vi "Is Air Pocket Part of Exterior Air Way.vi"(4 "Lava Droplets":set{cluster{"X":i32, "Y":i32, "Z":i32}}(c389), 5 "Extreme Planes":cluster{"X":i32[], "Y":i32[], "Z":i32[]}, 6 "Possible Directions":cluster{"X":i32, "Y":i32, "Z":i32}[](array[cluster]), 7 "Air Pockets Connected to Exterior Surface in":set{cluster{"X":i32, "Y":i32, "Z":i32}}(c389), 9 "Locations in Search in":set{cluster{"X":i32, "Y":i32, "Z":i32}}(c389), 10 "Location":cluster{"X":i32, "Y":i32, "Z":i32}) -> (0 "Air Pockets Connected to Exterior Surface out":set{cluster{"X":i32, "Y":i32, "Z":i32}}(c389), 2 "Locations in Search out":set{cluster{"X":i32, "Y":i32, "Z":i32}}(c389), 3 "Air Pocket Connected to Exterior Air way ?":bool)   [LabVIEW 2020, in "AoC 2022.lvlib"]
uses:
  AoC 2022.lvlib
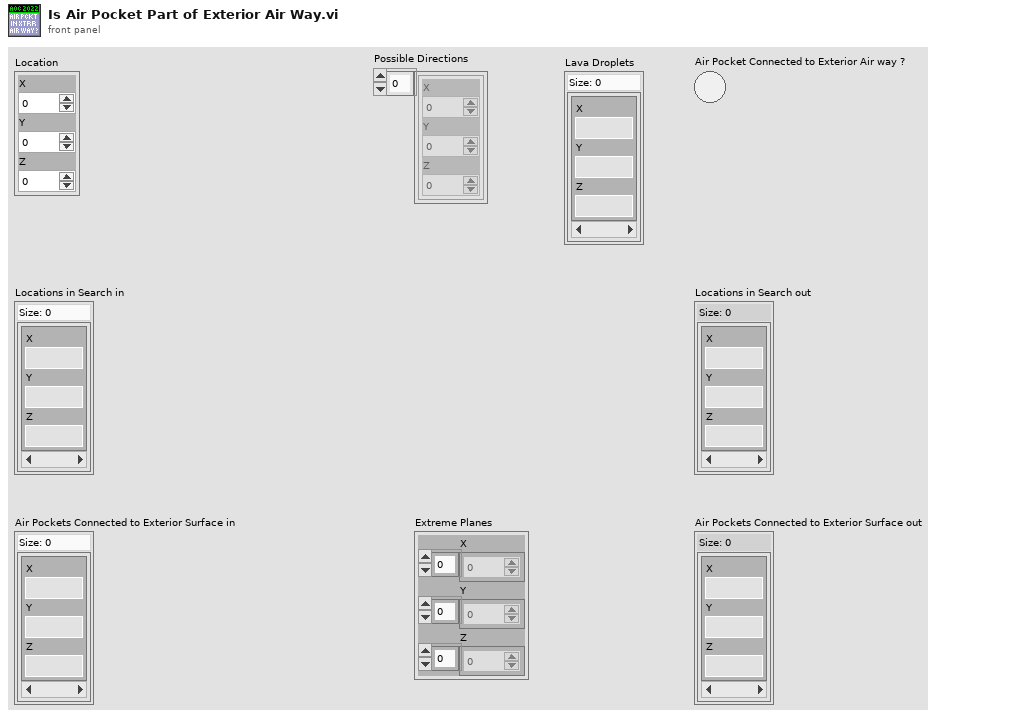
[diagram p1: front panel]
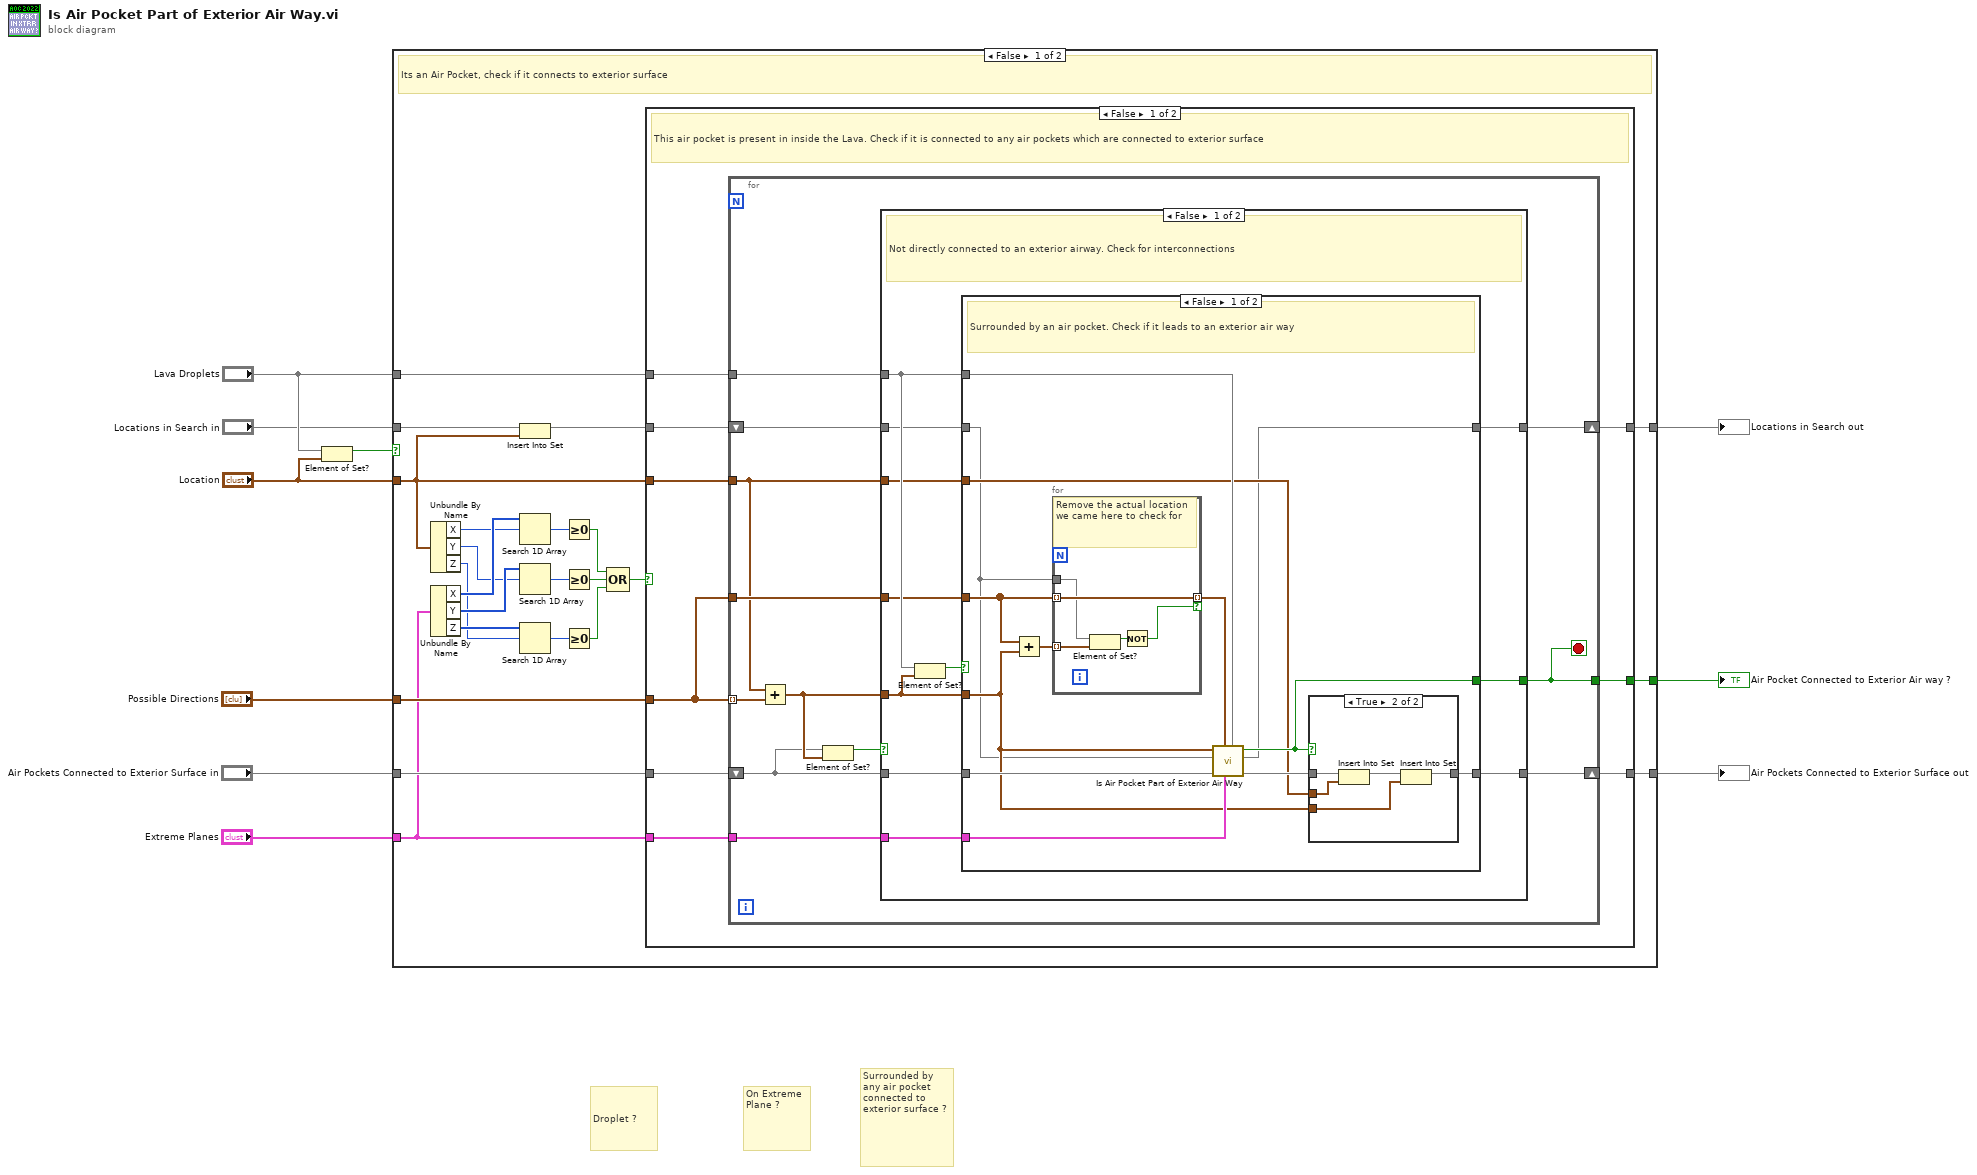
[diagram p0: block diagram]
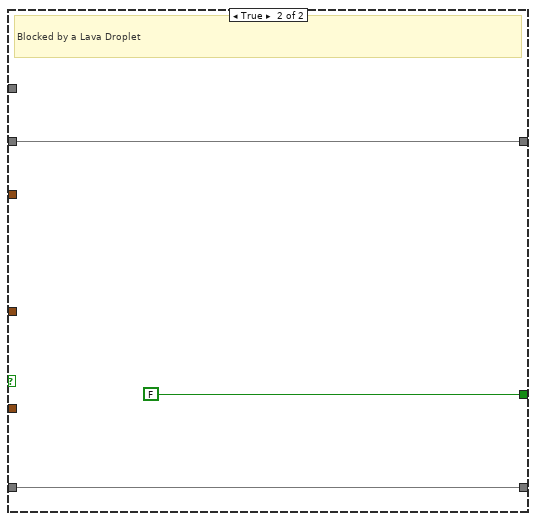
[diagram p3: hidden frame]
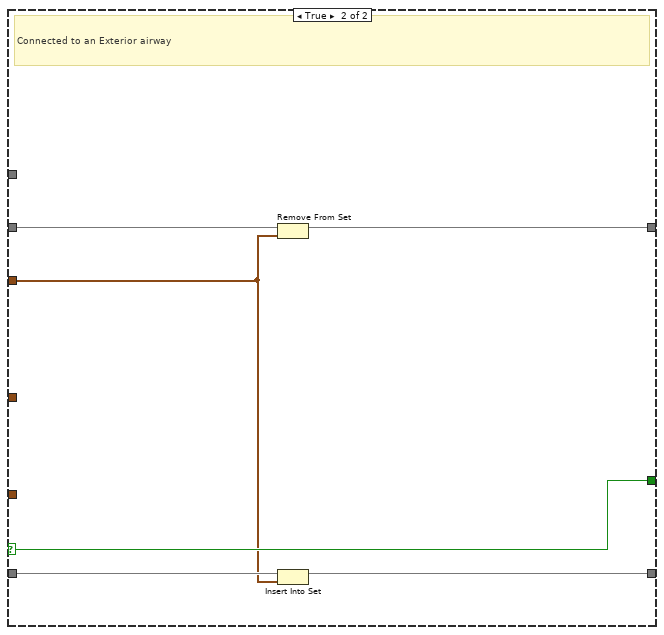
[diagram p4: hidden frame]
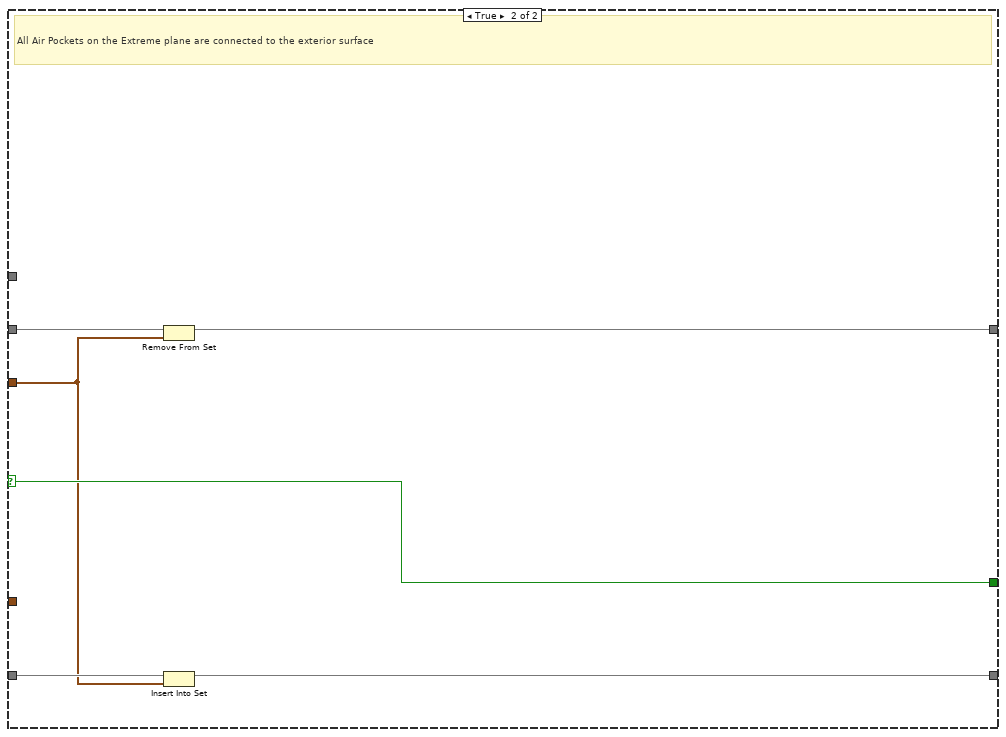
[diagram p5: hidden frame]
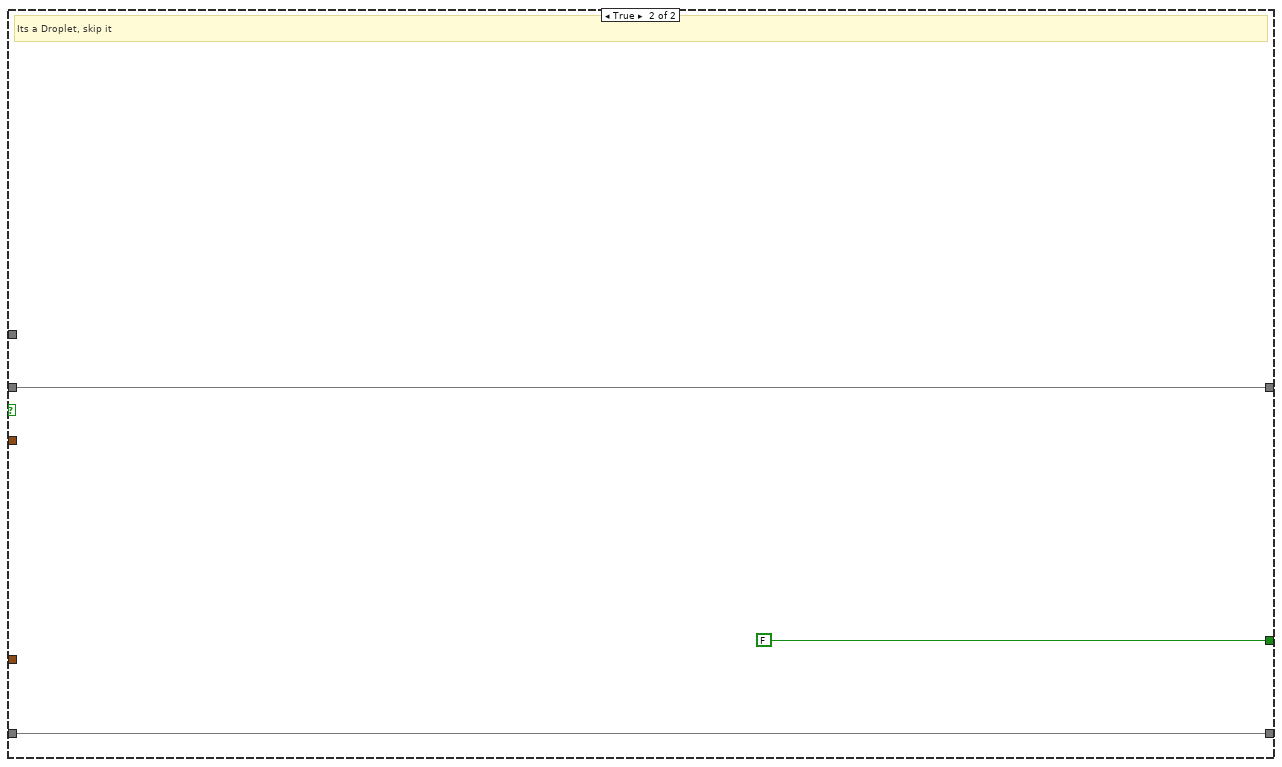
[diagram p6: hidden frame]
diagram:
  # "Surrounded by any air pocket connected to exterior surface ?"
  # "On Extreme Plane ?"
  # "Droplet ?"
  n1 = Element of Set?(10:"Location", 11:"Lava Droplets") -> (3:w8:bool)
  n2 = case shown="False" w8 {
    tunnel: "Air Pockets Connected to Exterior Surface in" -> [w33 w107]
    tunnel: [w32 w107] -> w4
    tunnel: "Possible Directions" -> [w31 _]
    tunnel: "Lava Droplets" -> [w30 _]
    tunnel: "Location" -> [w12 _]
    tunnel: "Extreme Planes" -> [w15 _]
    tunnel: [w16 FALSE] -> w10
    tunnel: "Locations in Search in" -> [w14 w105]
    tunnel: [w11 w105] -> w1
    frame False {
      # "Its an Air Pocket, check if it connects to exterior surface"
      n3 = Unbundle By Name(w12) -> ("X"=w28:i32, "Y"=w26:i32, "Z"=w24:i32)
      n4 = Unbundle By Name(w15) -> ("X"=w29:i32[], "Y"=w27:i32[], "Z"=w25:i32[])
      n5 = Insert Into Set(10:w12, 11:w14) -> (3:w13:set{cluster{"X":i32, "Y":i32, "Z":i32}})  [unwired: 1 out]
      n6 = Search 1D Array(1D array=w29, element=w28) -> (index of element=w23:i32)  [unwired: 1 in]
      n7 = Search 1D Array(1D array=w27, element=w26) -> (index of element=w21:i32)  [unwired: 1 in]
      n8 = Search 1D Array(1D array=w25, element=w24) -> (index of element=w22:i32)  [unwired: 1 in]
      n9 = Greater Or Equal To 0?(x=w23) -> (x >= 0?=w20:bool)
      n10 = Greater Or Equal To 0?(x=w21) -> (x >= 0?=w19:bool)
      n11 = Greater Or Equal To 0?(x=w22) -> (x >= 0?=w18:bool)
      n12 = Compound Arithmetic op=OR(w20, w19, w18) -> (w17:bool)
      n13 = case shown="False" w17 {
        selector: w17 -> [_ w102]
        tunnel: w33 -> [w42 w104]
        tunnel: [w41 w103] -> w32
        tunnel: w31 -> [w36 _]
        tunnel: w30 -> [w40 _]
        tunnel: w12 -> [w39 w99]
        tunnel: [w38 w102] -> w16
        tunnel: w15 -> [w37 _]
        tunnel: w13 -> [w35 w101]
        tunnel: [w34 w100] -> w11
        frame False {
          # "This air pocket is present in inside the Lava. Check if it is connected to any air pockets which are connected to exterior surface"
          n14 = for {
            tunnel: w39 -> [w45]
            shift-right: [w49] -> w41
            shift-left: w42 -> [w50]
            tunnel: w36 -> [w54] mode=indexing
            tunnel: w40 -> [w53]
            tunnel: [w48] -> w38
            tunnel: w37 -> [w47]
            tunnel: w36 -> [w46]
            shift-right: [w43] -> w34
            shift-left: w35 -> [w44]
            stop <- w48 stop-if-true
            n15 = Add(x=w45, y=w54) -> (x+y=w51:cluster{"X":i32, "Y":i32, "Z":i32})
            n16 = Element of Set?(10:w51, 11:w50) -> (3:w52:bool)
            n17 = case shown="False" w52 {
              selector: w52 -> [_ w98]
              tunnel: w53 -> [w60 _]
              tunnel: w51 -> [w58 _]
              tunnel: w50 -> [w64 w97]
              tunnel: [w65 w96] -> w49
              tunnel: [w62 w98] -> w48
              tunnel: w47 -> [w61 _]
              tunnel: w46 -> [w59 _]
              tunnel: w45 -> [w57 w93]
              tunnel: w44 -> [w56 w95]
              tunnel: [w55 w94] -> w43
              frame False {
                # "Not directly connected to an exterior airway. Check for interconnections"
                n18 = Element of Set?(10:w58, 11:w60) -> (3:w63:bool)
                n19 = case shown="False" w63 {
                  tunnel: [w71 w92] -> w65
                  tunnel: w64 -> [w77 w92]
                  tunnel: [w70 FALSE] -> w62
                  tunnel: w61 -> [w76 _]
                  tunnel: w60 -> [w78 _]
                  tunnel: w59 -> [w74 _]
                  tunnel: w58 -> [w68 _]
                  tunnel: w57 -> [w69 _]
                  tunnel: w56 -> [w67 w90]
                  tunnel: [w66 w90] -> w55
                  frame False {
                    # "Surrounded by an air pocket. Check if it leads to an exterior air way"
                    n20 = Add(x=w74, y=w68) -> (x+y=w75:cluster{"X":i32, "Y":i32, "Z":i32}[])
                    n21 = for {
                      tunnel: w75 -> [w88] mode=indexing
                      tunnel: w74 -> [w89] mode=indexing
                      tunnel: [w89] -> w73 mode=indexing if=w86
                      tunnel: w67 -> [w85]
                      # "Remove the actual location we came here to check for"
                      n22 = Element of Set?(10:w88, 11:w85) -> (3:w87:bool)
                      n23 = Not(x=w87) -> (.not. x?=w86:bool)
                    }
                    n24 = call "Is Air Pocket Part of Exterior Air Way.vi"("Lava Droplets"=w78, "Extreme Planes"=w76, "Possible Directions"=w73, "Air Pockets Connected to Exterior Surface in"=w77, "Locations in Search in"=w67, "Location"=w68) -> ("Air Pockets Connected to Exterior Surface out"=w72:set{cluster{"X":i32, "Y":i32, "Z":i32}}, "Locations in Search out"=w66:set{cluster{"X":i32, "Y":i32, "Z":i32}}, "Air Pocket Connected to Exterior Air way ?"=w70:bool)  [unwired: 2 in]
                    n25 = case shown="True" w70 {
                      tunnel: w72 -> [w79 w84]
                      tunnel: [w79 w82] -> w71
                      tunnel: w69 -> [_ w83]
                      tunnel: w68 -> [_ w80]
                      frame False {
                      }
                      frame True {
                        n26 = Insert Into Set(10:w83, 11:w84) -> (3:w81:set{cluster{"X":i32, "Y":i32, "Z":i32}})  [unwired: 1 out]
                        n27 = Insert Into Set(10:w80, 11:w81) -> (3:w82:set{cluster{"X":i32, "Y":i32, "Z":i32}})  [unwired: 1 out]
                      }
                    }
                  }
                  frame True {
                    # "Blocked by a Lava Droplet"
                  }
                }
              }
              frame True {
                # "Connected to an Exterior airway"
                n28 = Remove From Set(10:w93, 11:w95) -> (3:w94:set{cluster{"X":i32, "Y":i32, "Z":i32}})  [unwired: 1 out]
                n29 = Insert Into Set(10:w93, 11:w97) -> (3:w96:set{cluster{"X":i32, "Y":i32, "Z":i32}})  [unwired: 1 out]
              }
            }
          }
        }
        frame True {
          # "All Air Pockets on the Extreme plane are connected to the exterior surface"
          n30 = Remove From Set(10:w99, 11:w101) -> (3:w100:set{cluster{"X":i32, "Y":i32, "Z":i32}})  [unwired: 1 out]
          n31 = Insert Into Set(10:w99, 11:w104) -> (3:w103:set{cluster{"X":i32, "Y":i32, "Z":i32}})  [unwired: 1 out]
        }
      }
    }
    frame True {
      # "Its a Droplet, skip it"
    }
  }
  "Air Pocket Connected to Exterior Air way ?" <- w10
  "Air Pockets Connected to Exterior Surface out" <- w4
  "Locations in Search out" <- w1
